vi "超标留样启动.vi"(8 "error in (no error)":errorcluster) -> ()   [LabVIEW 2016, in "德润超标留样.lvlib"]
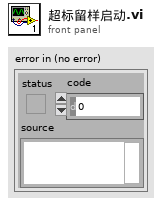
[diagram p1: front panel]
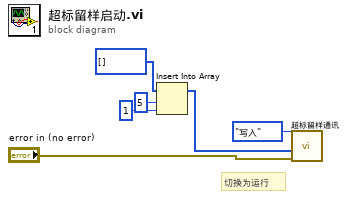
[diagram p0: block diagram]
diagram:
  # "切换为运行"
  n1 = Insert Into Array(array=u16[] [] ("values"), index=5 ("索引"), new element=u16 1 ("新元素/子数组")) -> (w1:u16[])
  n2 = call "超标留样通讯.vi"("Error in"="error in (no error)", "values"=w1, "starting address"=enum16{"打开串口", "写入", "读取", "关闭串口"}."写入" ("功能输入")) -> ()  [unwired: 5 in, 4 out]
